vi "SendTCPPackage.vi"(0 "connection ID":refnum<k5>, 1 "command":T1 items=["GarbageCollect", "GetAllObjects", "GetAllObjectsReply", "CleanUp", "G#Event", "RegisterClient", "GetAttributeValue", "GetAttributeValueReply", "GetClassAttributeValue", "GetClassAttributeValueReply", "GetToStringValue", "GetToStringValueReply", "GetClassHierarchy", "GetClassHierarchyReply", "Destroy", "RemoveClient"], 2 "data":string, 4 "timeout ms (200)":i32=200, 5 "error in (no error)":errorcluster) -> (19 "error out":errorcluster)   [LabVIEW 2017, in "G#RemoteProxy.lvclass"]
doc: "Sends an UDP package."
uses:
  G#RemoteProxy.lvclass
  G#DebugServer/utils/TCPCommand.ctl
  G#DebugServer/G#DebugServer.lvclass
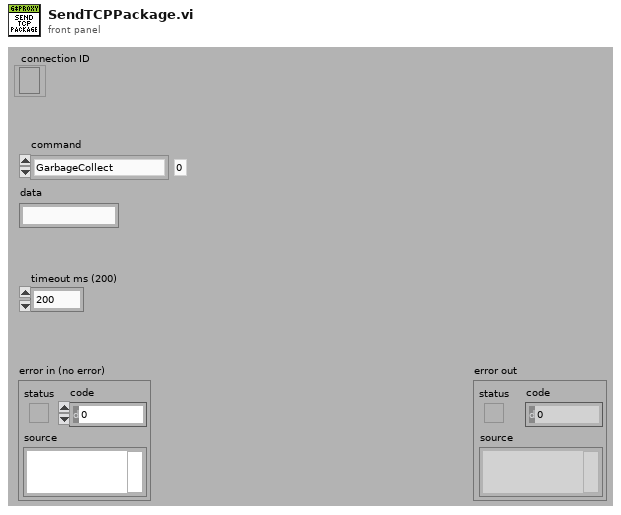
[diagram p1: front panel]
types:
  T1 = typedef "G#DebugServer.lvclass/TCPCommand.ctl" = u8
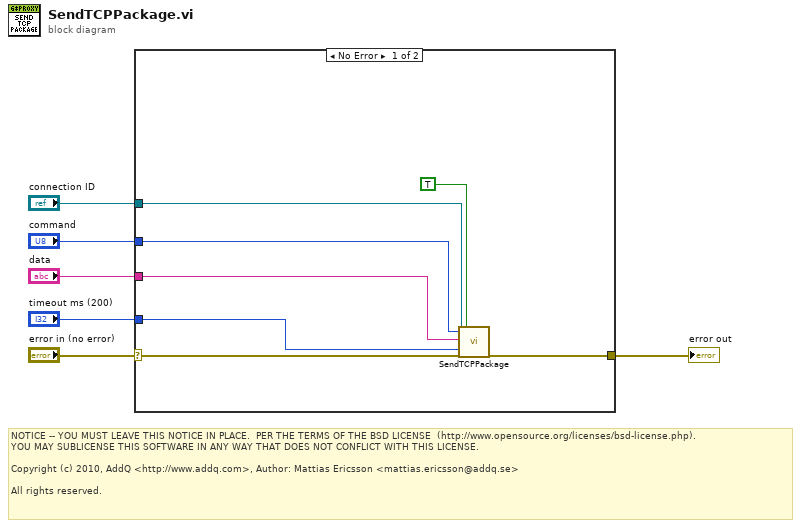
[diagram p0: block diagram]
diagram:
  # "NOTICE -- YOU MUST LEAVE THIS NOTICE IN PLACE.  PER THE TERMS OF THE BSD LICENSE  (http://www.opensource.org/licenses/bsd-license.php).\nYOU MAY SUBLICENSE THIS SOFTWARE IN ANY WAY THAT DOES NOT CONFLICT WITH THIS LICENSE.\n\nCopyright (c) 2010, AddQ <http://www.addq.com>, Author: Mattias Ericsson <mattias.ericsson@addq.se>\n\nAll rights reserved."
  n1 = case shown="No Error" "error in (no error)" {
    selector: "error in (no error)" -> [w13 w14]
    tunnel: [w10 w14] -> w5
    tunnel: "connection ID" -> [w9 _]
    tunnel: "command" -> [w12 _]
    tunnel: "data" -> [w11 _]
    tunnel: "timeout ms (200)" -> [w8 _]
    frame No Error {
      n2 = call "SendTCPPackage.vi"("connection ID"=w9, "command"=w12, "data"=w11, "timeout ms (200)"=w8, "error in (no error)"=w13, "enabled"=TRUE ("Enabled")) -> ("error out"=w10:errorcluster)  [unwired: 13 in]
    }
    frame Error {
    }
  }
  "error out" <- w5
